vi "Sweep.vi"(8 "error in (no error)":errorcluster, 11 "Spectrum Recorder in":refnum<class "Spectrum Recorder.lvclass">) -> (0 "error out":errorcluster, 3 "Spectrum Recorder out":refnum<class "Spectrum Recorder.lvclass">)   [LabVIEW 2016, in "Spectrum Recorder.lvclass"]
uses:
  Spectrum Recorder.lvclass
  Spectrum Recorder.lvclass/Spectrum Recorder.ctl
  Red Pitaya/RP Core/RP Transceiver/RP Transceiver.lvclass
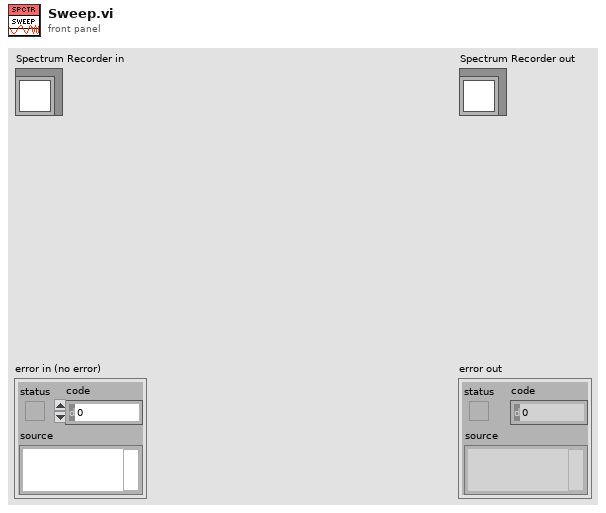
[diagram p1: front panel]
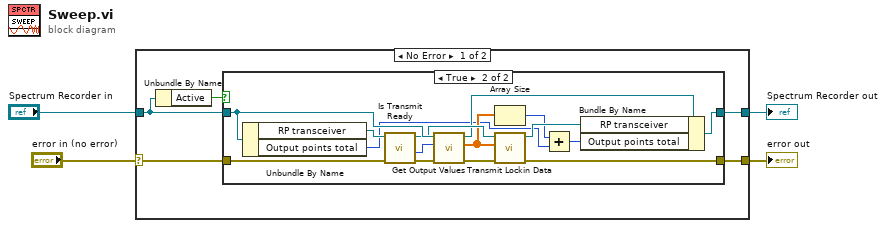
[diagram p0: block diagram]
diagram:
  n1 = case shown="No Error" "error in (no error)" {
    selector: "error in (no error)" -> [w6 w28]
    tunnel: [w5 w28] -> w3
    tunnel: [w7 w27] -> w1
    tunnel: "Spectrum Recorder in" -> [w8 w27]
    frame No Error {
      n2 = Unbundle By Name(w8) -> ("Active"=w9:bool)
      n3 = case shown="True" w9 {
        tunnel: w8 -> [w11 w24]
        tunnel: w6 -> [w10 w25]
        tunnel: [w11 w17] -> w7
        tunnel: [w10 w16] -> w5
        frame False {
        }
        frame True {
          n4 = Unbundle By Name(w24) -> ("RP transceiver"=w26:refnum<class "RP Transceiver.lvclass">, "Output points total"=w13:i64)
          n5 = call-dynamic "Is Transmit Ready.vi"("error in (no error)"=w25, "RP Instrument in"=w26) -> ("error out"=w22:errorcluster, "Unused buffer"=w23:i32, "RP Instrument out"=w21:refnum<class "RP Transceiver.lvclass">)  [unwired: 6 in, 1 out]
          n6 = call-dynamic "Get Output Values.vi"("error in (no error)"=w22, "Number of points"=w23, "Spectrum Recorder in"=w24) -> ("error out"=w20:errorcluster, "Output values"=w15:dbl[], "Spectrum Recorder out"=w19:refnum<class "Spectrum Recorder.lvclass">)  [unwired: 6 in]
          n7 = Array Size(array=w15) -> (size(s)=w14:i32)
          n8 = call-dynamic "Transmit Lockin Data.vi"("error in (no error)"=w20, "Data"=w15, "RP Transceiver in"=w21) -> ("error out"=w16:errorcluster, "RP Transceiver out"=w18:refnum<class "RP Transceiver.lvclass">)  [unwired: 6 in, 1 out]
          n9 = Add(x=w14, y=w13) -> (x+y=w12:i64)
          n10 = Bundle By Name(cluster=w19, "RP transceiver"=w18, "Output points total"=w12) -> (w17:refnum<class "Spectrum Recorder.lvclass">)
        }
      }
    }
    frame Error {
    }
  }
  "error out" <- w3
  "Spectrum Recorder out" <- w1
